vi "Read RP Instrument.lvclass.vi"(8 "error in (no error)":errorcluster, 11 "Red Pitaya Digitizer in":refnum<class "Red Pitaya Recorder.lvclass">) -> (0 "error out":errorcluster, 2 "RP Instrument.lvclass":refnum<class "RP Instrument.lvclass">, 3 "Red Pitaya Digitizer out":refnum<class "Red Pitaya Recorder.lvclass">)   [LabVIEW 2015, in "Red Pitaya Recorder.lvclass"]
uses:
  Red Pitaya Recorder.lvclass
  NHMFL_Core/Libraries/Red Pitaya/RP Core/RP Instrument/RP Instrument.lvclass
  Red Pitaya Recorder.lvclass/Red Pitaya Recorder.ctl
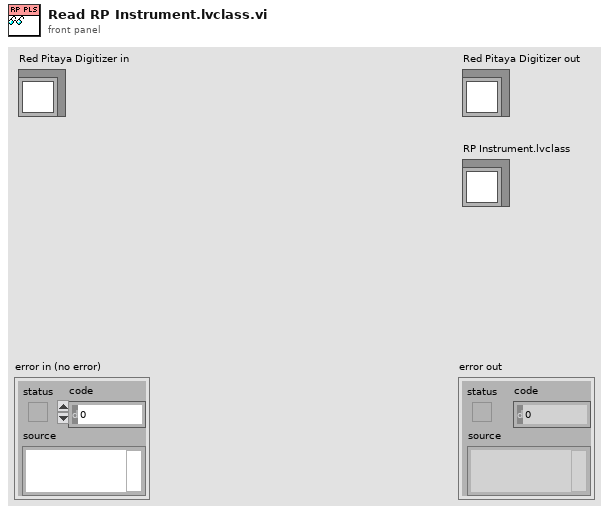
[diagram p1: front panel]
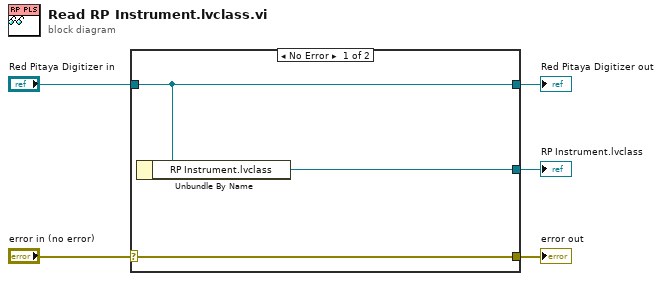
[diagram p0: block diagram]
diagram:
  n1 = case shown="No Error" "error in (no error)" {
    selector: "error in (no error)" -> [w8 w9]
    tunnel: [w8 w9] -> w4
    tunnel: [w7 w10] -> w2
    tunnel: "Red Pitaya Digitizer in" -> [w7 w10]
    tunnel: [w6 _] -> w1
    frame No Error {
      n2 = Unbundle By Name(w7) -> ("RP Instrument.lvclass"=w6:refnum<class "RP Instrument.lvclass">)
    }
    frame Error {
    }
  }
  "error out" <- w4
  "Red Pitaya Digitizer out" <- w2
  "RP Instrument.lvclass" <- w1
